vi "hne_Page State.vi"(6 "Page Operation":T1=enum."Set Next", 7 "Initial Page":string, 10 "Max page history length":i32, 11 "Next Page":string) -> (3 "Next Page":string)   [LabVIEW 2013]
doc: "This is the Page manager that keeps the pages history."
uses:
  TypeDefs/Page Operation.ctl
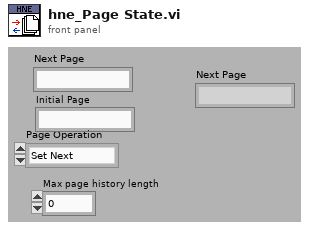
[diagram p1: front panel]
types:
  T1 = typedef "Page Operation.ctl" = enum16{"Init", "Set Next", "Get Next", "Back"}
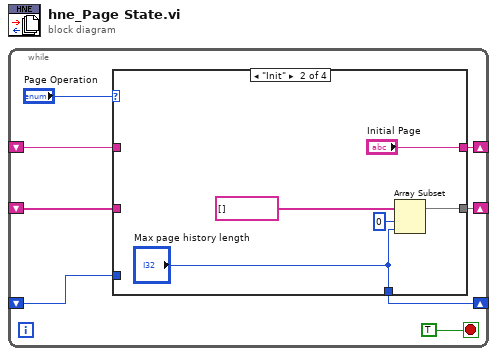
[diagram p0: block diagram]
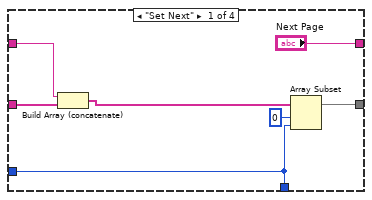
[diagram p2: hidden frame]
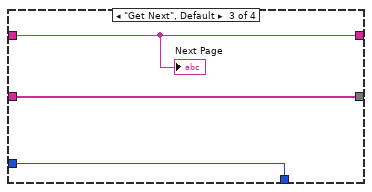
[diagram p3: hidden frame]
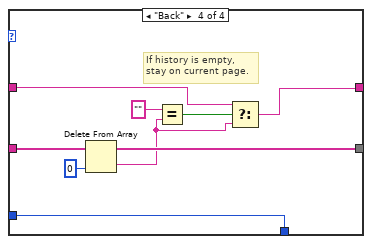
[diagram p4: hidden frame]
diagram:
  n1 = while {
    shift-right: [w7] -> _
    shift-left: _ -> [w6]
    shift-right: [w5] -> _
    shift-left: _ -> [w4]
    shift-right: [w2] -> _
    shift-left: _ -> [w1]
    stop <- TRUE stop-if-true
    n2 = case shown="\"Init\"" "Page Operation" {
      tunnel: [w14 w19 w22 w30] -> w7
      tunnel: w6 -> [w12 _ w22 w31]
      tunnel: ["Next Page" "Initial Page" w23 w25] -> w5
      tunnel: w4 -> [w11 _ w23 w27]
      tunnel: [w10 "Max page history length" w21 w24] -> w2
      tunnel: w1 -> [w10 _ w21 w24]
      frame "Set Next" {
        n3 = Build Array (concatenate)(w11, w12) -> (w9:string[])
        n4 = Array Subset(array=w9, index=0, length=w10) -> (w14:string[])
      }
      frame "Init" {
        n5 = Array Subset(array=string[] [] ("Page History"), index=0, length="Max page history length") -> (w19:string[])
      }
      frame "Get Next", Default {
        "Next Page" <- w23
      }
      frame "Back" {
        # "If history is empty,\nstay on current page."
        n6 = Delete From Array(array=w31, index=0) -> (deleted portion=w26:string, array with subset deleted=w30:string[])  [unwired: 1 in]
        n7 = Equal?(x="" ("y"), y=w26) -> (x = y?=w28:bool)
        n8 = Select(t=w27, s=w28, f=w26) -> (s? t:f=w25:string)
      }
    }
  }
